vi "PostCopyScripting.vi"(10 "MetaDataObj":refnum<class "MetaDataObj.lvclass">, 11 "User Project":refnum<vi>) -> ()   [LabVIEW 2013, in "FixedChannelTBModuleDecideFeatures.lvclass"]
uses:
  FixedChannelTBModuleDecideFeatures.lvclass
  <resource>/dialog/NewProjectWizard/MetaDataObj/MetaDataObj.lvclass
  <vilib>/NI/DCAF/Tag Editor Core/control module/script/Controls/processing script control.ctl
  <vilib>/NI/DCAF/Tag Editor Core/control module/script/Controls/output script control.ctl
  <vilib>/NI/DCAF/Tag Editor Core/control module/script/Controls/input script control.ctl
  FixedChannelTBModuleDecideFeatures.lvclass/FixedChannelTBModuleDecideFeatures.ctl
  Read component name.vi
  Read Channel Specification.vi
  <vilib>/NI/DCAF/Tag Editor Core/control module/script/control module data interface generator.lvlib
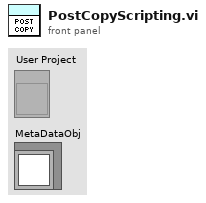
[diagram p1: front panel]
types:
  T1 = typedef "control module data interface generator.lvlib/input script control.ctl" = cluster{"enable?":bool, "Data Interface VI (blank=input to tag bus.vi)":string, "reverse?":bool, "Reverse Interface VI (blank=input from tag bus.vi)":string}
  T2 = typedef "control module data interface generator.lvlib/output script control.ctl" = cluster{"enable?":bool, "Data Interface VI (blank=tag bus to outputs.vi)":string, "Reverse Interface VI (blank=tag bus from outputs.vi)":string, "reverse?":bool}
  T3 = typedef "control module data interface generator.lvlib/processing script control.ctl" = cluster{"param?":bool, "Parameter Data Interface VI (blank=tag bus to parameters.vi)":string, "Result Data Interface VI (blank=results to tag bus.vi)":string, "reverse param?":bool, "Rev. Result Interface VI (blank=results from tag bus.vi)":string, "Rev. Parameter Interface VI (blank=tag bus from parameters.vi)":string, "result?":bool, "reverse result?":bool}
  T4 = typedef "FixedChannelTBModuleDecideFeatures.lvclass/channel configuration.ctl" = cluster{"Name":string, "channel classification":T5, "data type":T6}
  T5 = typedef "TBM channel.lvclass/channel classification.ctl" = enum16{"input data", "output data", "processing parameter", "processing result"}
  T6 = typedef "tag bus.lvlib/tag descriptor.lvclass/Data Type.ctl" = enum16{"Double", "Single", "I64", "I32", "I16", "I8", "U64", "U32", "U16", "U8", "Boolean", "String", "Array of Double", "Array of Single", "Array of I64", "Array of I32", "Array of I16", "Array of I8", "Array of U64", "Array of U32", "Array of U16", "Array of U8", "Array of Boolean", "Array of String"}
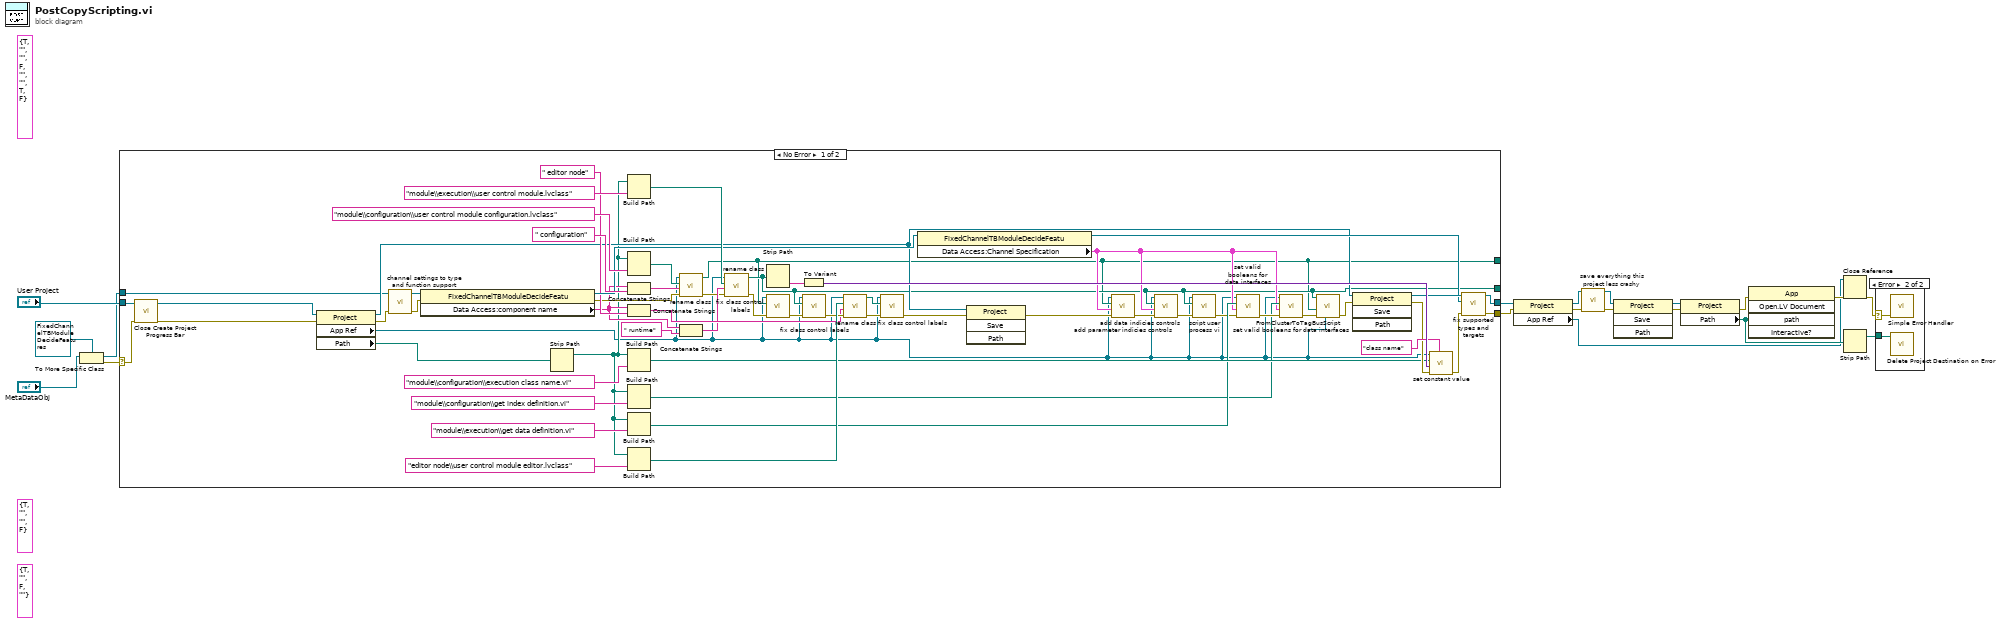
[diagram p0: block diagram]
diagram:
  (unwired) T1 {"enable?"=TRUE, "Data Interface VI (blank=input to tag bus.vi)"="", "reverse?"=FALSE, "Reverse Interface VI (blank=input from tag bus.vi)"=""} ("input")
  (unwired) T2 {"enable?"=TRUE, "Data Interface VI (blank=tag bus to outputs.vi)"="", "Reverse Interface VI (blank=tag bus from outputs.vi)"="", "reverse?"=FALSE} ("output")
  (unwired) T3 {"param?"=TRUE, "Parameter Data Interface VI (blank=tag bus to parameters.vi)"="", "Result Data Interface VI (blank=results to tag bus.vi)"="", "reverse param?"=FALSE, "Rev. Result Interface VI (blank=results from tag bus.vi)"="", "Rev. Parameter Interface VI (blank=tag bus from parameters.vi)"="", "result?"=TRUE, "reverse result?"=FALSE} ("process")
  n1 = To More Specific Class(target class=refnum<class "FixedChannelTBModuleDecideFeatures.lvclass"> refnum ("DecideProjectFeatures.lvclass"), reference="MetaDataObj") -> (specific class reference=w10:refnum<class "FixedChannelTBModuleDecideFeatures.lvclass">, error out=w17:errorcluster)  [unwired: 1 in]
  n2 = case shown="No Error" w17 {
    selector: w17 -> [w36 w79]
    tunnel: [w58 w80] -> w3
    tunnel: "User Project" -> [w37 w80]
    tunnel: [w59 w79] -> w2
    tunnel: w10 -> [w43 _]
    tunnel: [w24 _] -> _
    tunnel: [w23 _] -> _
    frame No Error {
      n3 = call <resource>:"Close Create Project Progress Bar.vi"("error in (no error)"=w36, "Project"=w37) -> ("error out"=w35:errorcluster, "dup Project"=w34:refnum<vi>)  [unwired: 8 in]
      n4 = property class="Project"(reference=w34, error in=w35) -> (reference out=w48:refnum<vi>, error out=w42:errorcluster, "App Ref"=w20:refnum<vi>, "Path"=w47:path)
      n5 = call "channel settings to type and function support.vi"("error in"=w42, "FixedChannelTBModuleDecideFeatures in"=w43) -> ("error out"=w45:errorcluster, "FixedChannelTBModuleDecideFeatures out"=w44:refnum<class "FixedChannelTBModuleDecideFeatures.lvclass">)  [unwired: 8 in]
      n6 = property class="FixedChannelTBModuleDecideFeatu"(reference=w44, error in=w45) -> (reference out=w74:refnum<class "FixedChannelTBModuleDecideFeatures.lvclass">, error out=w46:errorcluster, "Data Access:component name"=w39:string)
      n7 = Strip Path(path=w47) -> (stripped path=w26:path)  [unwired: 1 out]
      n8 = Build Path(base path=w26, name or relative path="module\\execution\\user control module.lvclass") -> (appended path=w76:path)
      n9 = Build Path(base path=w26, name or relative path="module\\configuration\\user control module configuration.lvclass") -> (appended path=w51:path)
      n10 = Concatenate Strings(w39, " configuration" ("string")) -> (w56:string)
      n11 = Concatenate Strings(w39, " editor node" ("string")) -> (w60:string)
      n12 = Build Path(base path=w26, name or relative path="module\\configuration\\execution class name.vi") -> (appended path=w41:path)
      n13 = Build Path(base path=w26, name or relative path="module\\configuration\\get index definition.vi") -> (appended path=w29:path)
      n14 = Build Path(base path=w26, name or relative path="module\\execution\\get data definition.vi") -> (appended path=w31:path)
      n15 = Build Path(base path=w26, name or relative path="editor node\\user control module editor.lvclass") -> (appended path=w65:path)
      n16 = call "rename class.vi"("error in"=w46, "new name"=w56, "class path"=w51, "Application in"=w20) -> ("error out"=w52:errorcluster, "New Library Path"=w23:path)  [unwired: 6 in]
      n17 = Concatenate Strings(w39, " runtime" ("string")) -> (w53:string)
      n18 = call "rename class.vi"("error in"=w52, "new name"=w53, "class path"=w76, "Application in"=w20) -> ("error out"=w68:errorcluster, "New Library Path"=w24:path)  [unwired: 6 in]
      n19 = Strip Path(path=w24) -> (name=w55:string)  [unwired: 1 out]
      n20 = call "fix class control labels.vi"("error in"=w68, "class to load"=w23, "Application in"=w20) -> ("error out"=w67:errorcluster)  [unwired: 8 in]
      n21 = To Variant(anything=w55) -> (Variant=w73:variant)
      n22 = call "fix class control labels.vi"("error in"=w67, "class to load"=w24, "Application in"=w20) -> ("error out"=w62:errorcluster)  [unwired: 8 in]
      n23 = call "rename class.vi"("error in"=w62, "new name"=w60, "class path"=w65, "Application in"=w20) -> ("error out"=w63:errorcluster, "New Library Path"=w64:path)  [unwired: 6 in]
      n24 = call "fix class control labels.vi"("error in"=w63, "class to load"=w64, "Application in"=w20) -> ("error out"=w38:errorcluster)  [unwired: 8 in]
      n25 = property class="FixedChannelTBModuleDecideFeatu"(reference=w74) -> (reference out=w50:refnum<class "FixedChannelTBModuleDecideFeatures.lvclass">, "Data Access:Channel Specification"=w28:T4[])  [unwired: 1 in, 1 out]
      n26 = invoke class="Project" method="Save"(reference=w48, error in=w38) -> (error out=w49:errorcluster)  [unwired: 2 in, 3 out]
      n27 = call "add parameter indicies controls.vi"("error in"=w49, "Channels to create"=w28, "cfg class path"=w23, "Application in"=w20) -> ("error out"=w40:errorcluster)  [unwired: 7 in]
      n28 = call "add data indicies controls.vi"("error in"=w40, "Channels to create"=w28, "runtime class path"=w24, "Application in"=w20) -> ("error out"=w25:errorcluster)  [unwired: 6 in, 1 out]
      n29 = call "script user process vi.vi"("error in"=w25, "runtime class path in"=w24, "Application in"=w20) -> ("error out"=w27:errorcluster)  [unwired: 8 in]
      n30 = call "set valid booleans for data interfaces.vi"("error in"=w27, "Channel Specification"=w28, "vi path"=w31, "Application in"=w20) -> ("error out"=w30:errorcluster)  [unwired: 7 in]
      n31 = call "set valid booleans for data interfaces.vi"("error in"=w30, "Channel Specification"=w28, "vi path"=w29, "Application in"=w20) -> ("error out"=w22:errorcluster)  [unwired: 7 in]
      n32 = call <vilib>:"FromClusterToTagBusScript.vi"("application reference (local)"=w20, "error in"=w22, "configuration class path"=w23, "runtime class path"=w24) -> ("error out"=w21:errorcluster)  [unwired: 7 in]
      n33 = invoke class="Project" method="Save"(reference=w48, error in=w21) -> (reference out=w69:refnum<vi>, error out=w70:errorcluster)  [unwired: 2 in, 2 out]
      n34 = call "set constant value.vi"("control name"="class name", "error in"=w70, "data to set"=w73, "vi path"=w41, "Application in"=w20) -> ("error out"=w57:errorcluster)  [unwired: 6 in]
      n35 = call "fix supported types and targets.vi"("error in"=w57, "DecideProjectFeatures in"=w50, "User Project in"=w69) -> ("error out"=w59:errorcluster, "User Project out"=w58:refnum<vi>)  [unwired: 7 in]
    }
    frame Error {
    }
  }
  n36 = property class="Project"(reference=w3, error in=w2) -> (reference out=w7:refnum<vi>, error out=w8:errorcluster, "App Ref"=w6:refnum<vi>)
  n37 = call "save everything this project less crashy.vi"("error in"=w8, "Project in"=w7) -> ("error out"=w4:errorcluster, "Project out"=w9:refnum<vi>)  [unwired: 8 in]
  n38 = invoke class="Project" method="Save"(reference=w9, error in=w4) -> (reference out=w13:refnum<vi>, error out=w14:errorcluster)  [unwired: 2 in, 2 out]
  n39 = property class="Project"(reference=w13, error in=w14) -> (error out=w16:errorcluster, "Path"=w11:path)  [unwired: 1 out]
  n40 = invoke class="App" method="Open.LV Document"(error in=w16, "path"=w11) -> (error out=w15:errorcluster)  [unwired: 3 in, 4 out]
  n41 = Close Reference(reference=w6, error in (no error)=w15) -> (error out=w1:errorcluster)
  n42 = Strip Path(path=w11) -> (stripped path=w5:path)  [unwired: 1 out]
  n43 = case shown="Error" w1 {
    selector: w1 -> [_ w81]
    tunnel: w5 -> [_ w82]
    frame No Error {
    }
    frame Error {
      n44 = call <vilib>:"Simple Error Handler.vi"("error in (no error)"=w81) -> ()  [unwired: 4 in, 5 out]
      n45 = call <resource>:"Delete Project Destination on Error.vi"("Project Destination Root"=w82) -> ()  [unwired: 11 in]
    }
  }
